vi "Convert Error Code & Message to Error Cluster.vi"(0 "Error Code (no error: 0)":i32, 1 "Error Message":string) -> (2 "Error Out":errorcluster)   [LabVIEW 2021, in "Error.lvlib"]
uses:
  <vilib>/Utility/error.llb/DialogType.ctl
  Error.lvlib
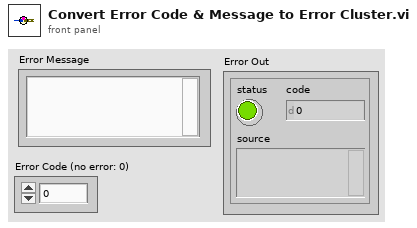
[diagram p1: front panel]
types:
  T1 = typedef "DialogType.ctl" = u16
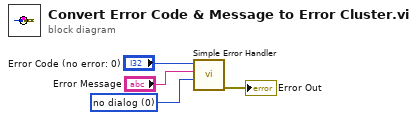
[diagram p0: block diagram]
diagram:
  w2 = T1 0 items=["no dialog", "OK message", "continue or stop message", "OK message + warnings", "continue/stop + warnings"] ("type of dialog (OK msg:1)")
  n1 = call <vilib>:"Simple Error Handler.vi"("error code (no error:0)"="Error Code (no error: 0)", "error source (\" \")"="Error Message", "type of dialog (OK msg:1)"=w2) -> ("error out"=→"Error Out":errorcluster)  [unwired: 2 in, 4 out]
